vi "getAllTicks.vi"(8 "error in (no error)":errorcluster, 11 "DeviceArray in":refnum<class "DeviceArray.lvclass">) -> (0 "error out":errorcluster, 2 "scriptEventListArray":refnum<class "ScriptEventList.lvclass">[](array[class]), 3 "DeviceArray out":refnum<class "DeviceArray.lvclass">)   [LabVIEW 2009, in "Tools.lvlib" / "DatabaseHelpers.lvlib" / "DeviceArray.lvclass"]
uses:
  DeviceArray.lvclass
  Scripting/ScriptingEvent/ScriptEventList/ScriptEventList.lvclass
  DeviceArray.lvclass/DeviceArray.ctl
  device/device.lvclass
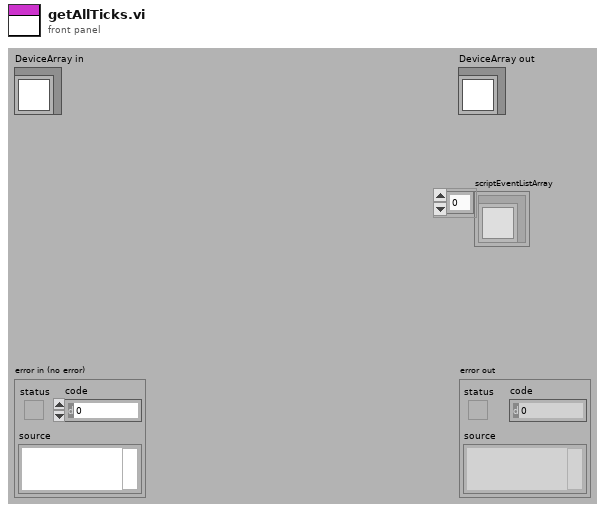
[diagram p1: front panel]
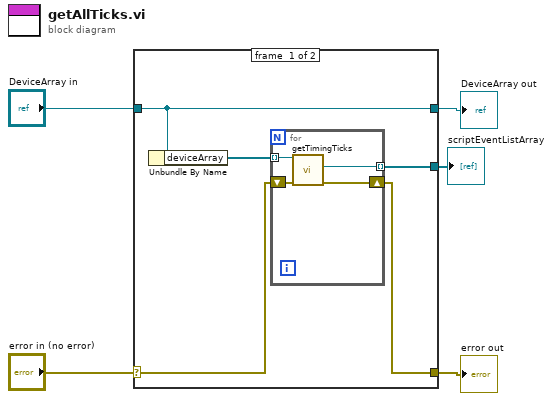
[diagram p0: block diagram]
diagram:
  n1 = case shown="No Error" "error in (no error)" {
    selector: "error in (no error)" -> [w8 w16]
    tunnel: [w6 w16] -> w4
    tunnel: [w10 w15] -> w2
    tunnel: "DeviceArray in" -> [w10 w15]
    tunnel: [w7 _] -> w1
    frame #0 {
      n2 = Unbundle By Name(w10) -> ("deviceArray"=w9:refnum<class "device.lvclass">[])
      n3 = for {
        tunnel: w9 -> [w14] mode=indexing
        tunnel: [w11] -> w7 mode=indexing
        shift-right: [w12] -> w6
        shift-left: w8 -> [w13]
        n4 = call "getTimingTicks.vi"("error in (no error)"=w13, "device.lvclass in"=w14) -> ("error out"=w12:errorcluster, "timingTicks"=w11:refnum<class "ScriptEventList.lvclass">)  [unwired: 7 in, 1 out]
      }
    }
    frame #1 {
    }
  }
  "error out" <- w4
  "DeviceArray out" <- w2
  "scriptEventListArray" <- w1
